vi "AI-Process Output Data.vi"(8 "error in (no error)":errorcluster, 11 "AI-Data In":T1(array[cluster])) -> (0 "error out":errorcluster, 3 "AI-Data Out":T2(array[cluster]))   [LabVIEW 2021]
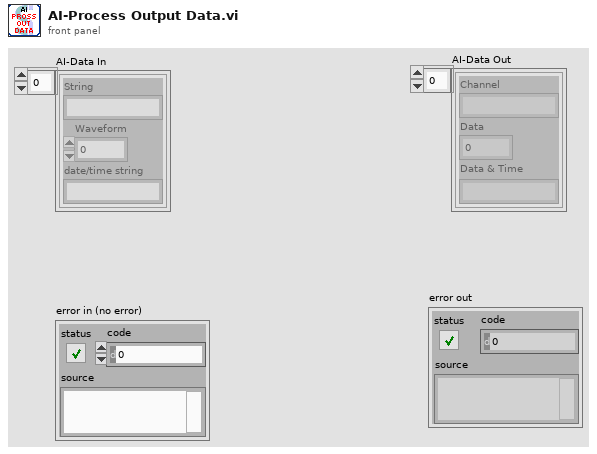
[diagram p1: front panel]
types:
  T1 = cluster{"String":string, "Waveform":dbl, "date/time string":string}[]
  T2 = cluster{"Channel":string, "Data":dbl, "Data & Time":string}[]
  T3 = cluster{"Channel":string, "Data":dbl, "Data & Time":string}
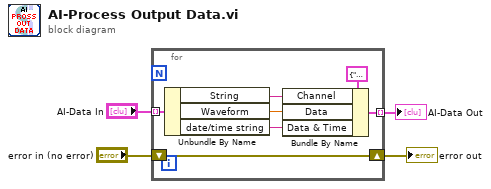
[diagram p0: block diagram]
diagram:
  n1 = for {
    tunnel: "AI-Data In" -> [w11] mode=indexing
    shift-right: [w6] -> w4
    shift-left: "error in (no error)" -> [w6]
    tunnel: [w5] -> w2 mode=indexing
    n2 = Unbundle By Name(w11) -> ("String"=w10:string, "Waveform"=w9:dbl, "date/time string"=w8:string)
    n3 = Bundle By Name(cluster=T3 {"Channel"="", "Data"=0.0, "Data & Time"=""} ("Cluster"), "Channel"=w10, "Data"=w9, "Data & Time"=w8) -> (w5:T3)
  }
  "error out" <- w4
  "AI-Data Out" <- w2
